vi "Address Space Size.vi"(2 "Oscillator":refnum<class "Oscillator.lvclass">) -> (6 "size":u32)   [LabVIEW 2017, in "Oscillator.lvlib" / "Oscillator.lvclass"]
uses:
  Oscillator.lvclass
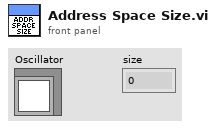
[diagram p1: front panel]
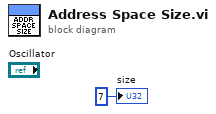
[diagram p0: block diagram]
diagram:
  "size" <- u32 7 ("size")
